vi "RunTimeMenuUI.vi"() -> ()   [LabVIEW 2015, in "RunTimeMenuItem.lvclass"]
uses:
  RunTimeMenuItem.lvclass
  <vilib>/NI/Configuration Framework/Node/NodeRef.ctl
  <vilib>/NI/Configuration Framework/Node/NISE_CEF_Node.lvclass
  <vilib>/NI/AMC/Message Queue.ctl
  <vilib>/NI/AMC/Message.ctl
  <vilib>/NI/Tools/Keyed Array/KeyedArray.ctl
  <vilib>/NI/Configuration Framework/Node/UserEventRef.ctl
  <vilib>/NI/Configuration Framework/Controls/EventCluster.ctl
  RunTimeMenuItem.lvclass/RunTimeMenuItem.ctl
  Read Run Time Menu Properties.vi
  Write Run Time Menu Properties.vi
  <vilib>/NI/AMC/Create Single Message.vi
  <vilib>/NI/AMC/Update Message Routing Info.vi
  <vilib>/NI/AMC/Send Message.vi
  <vilib>/NI/AMC/AMC.lvlib
  Configuration Tool.lvlib
  <vilib>/NI/Tools/Keyed Array/Tools_KeyedArray.lvlib
  <vilib>/NI/Configuration Framework/NISE_CEF_TreeControl.lvlib
panel:
  in  "Min # Of Children":u32
  in  "Dependency Behavior":enum16{"Static", "Dynamic"}(ring)
  in  "Behavior":enum16{"Nothing", "Open Front Panel"}(ring)
  in  "Position":enum16{"Centered", "Mouse Pointer"}(ring)
  in  "Execution":enum16{"silent", "modal", "floating", "default"}(ring)
  in  "Menu Item Type":enum16{"Action", "VI", "Separator", "Custom"}(ring)
  in  "Host Path to Dependency File":path
  in  "Host Path to Menu VI":path
  in  "Host Path to Custom Menu Item":path
  in  "GUID":string="9b525fa0-4d4a-4ec1-902b-bfeef88ebbcc"
  in  "Name":string
  in  "user event":T1
  in  "main queue":T2
  in  "node ref":T3
  # "General Settings"
  # "Advanced Settings"
  # "Dependency File Settings"
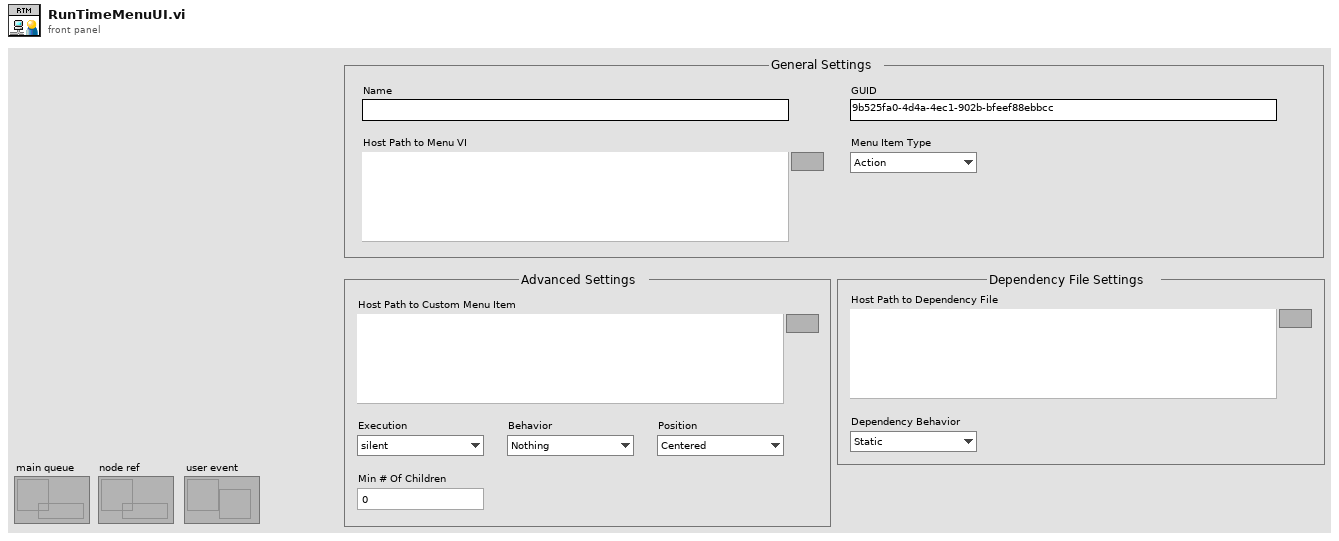
[diagram p1: front panel]
types:
  T1 = typedef "NISE_CEF_Node.lvclass/UserEventRef.ctl" = refnum<user-event>
  T2 = typedef "AMC.lvlib/Message Queue.ctl" = refnum<queue>
  T3 = typedef "NISE_CEF_Node.lvclass/NodeRef.ctl" = refnum<data-value>
  T4 = typedef "VeriStand Custom Device XML Parser.lvlib/RunTimeMenus Properties.ctl" = cluster{"GUID":string, "Execution":T5, "MinNrOfChilds":u32, "Name":string, "Item to Launch":T6, "Dependency":T7, "Custom Population":T6, "Menu Item Type":enum16{"Action", "VI", "Separator", "Custom"}, "Behavior":enum16{"Nothing", "Open Front Panel"}, "Position":enum16{"Centered", "Mouse Pointer"}}
  T5 = typedef "VeriStand Custom Device XML Parser.lvlib/Execution Types.ctl" = enum16{"silent", "modal", "floating", "default"}
  T6 = typedef "VeriStand Custom Device XML Parser.lvlib/Path Cluster.ctl" = cluster{"Path":path, "Path Type":enum16{"Absolute", "To Base", "To Common Doc Dir", "To Application Data Dir"}}
  T7 = typedef "VeriStand Custom Device XML Parser.lvlib/Dependency Properties.ctl" = cluster{"File Path Control":path, "Path Type":enum16{"Absolute", "To Base", "To Common Doc Dir", "To Application Data Dir"}, "Behavior":enum16{"Static", "Dynamic"}}
  T8 = enum16{"Absolute", "To Base", "To Common Doc Dir", "To Application Data Dir"}
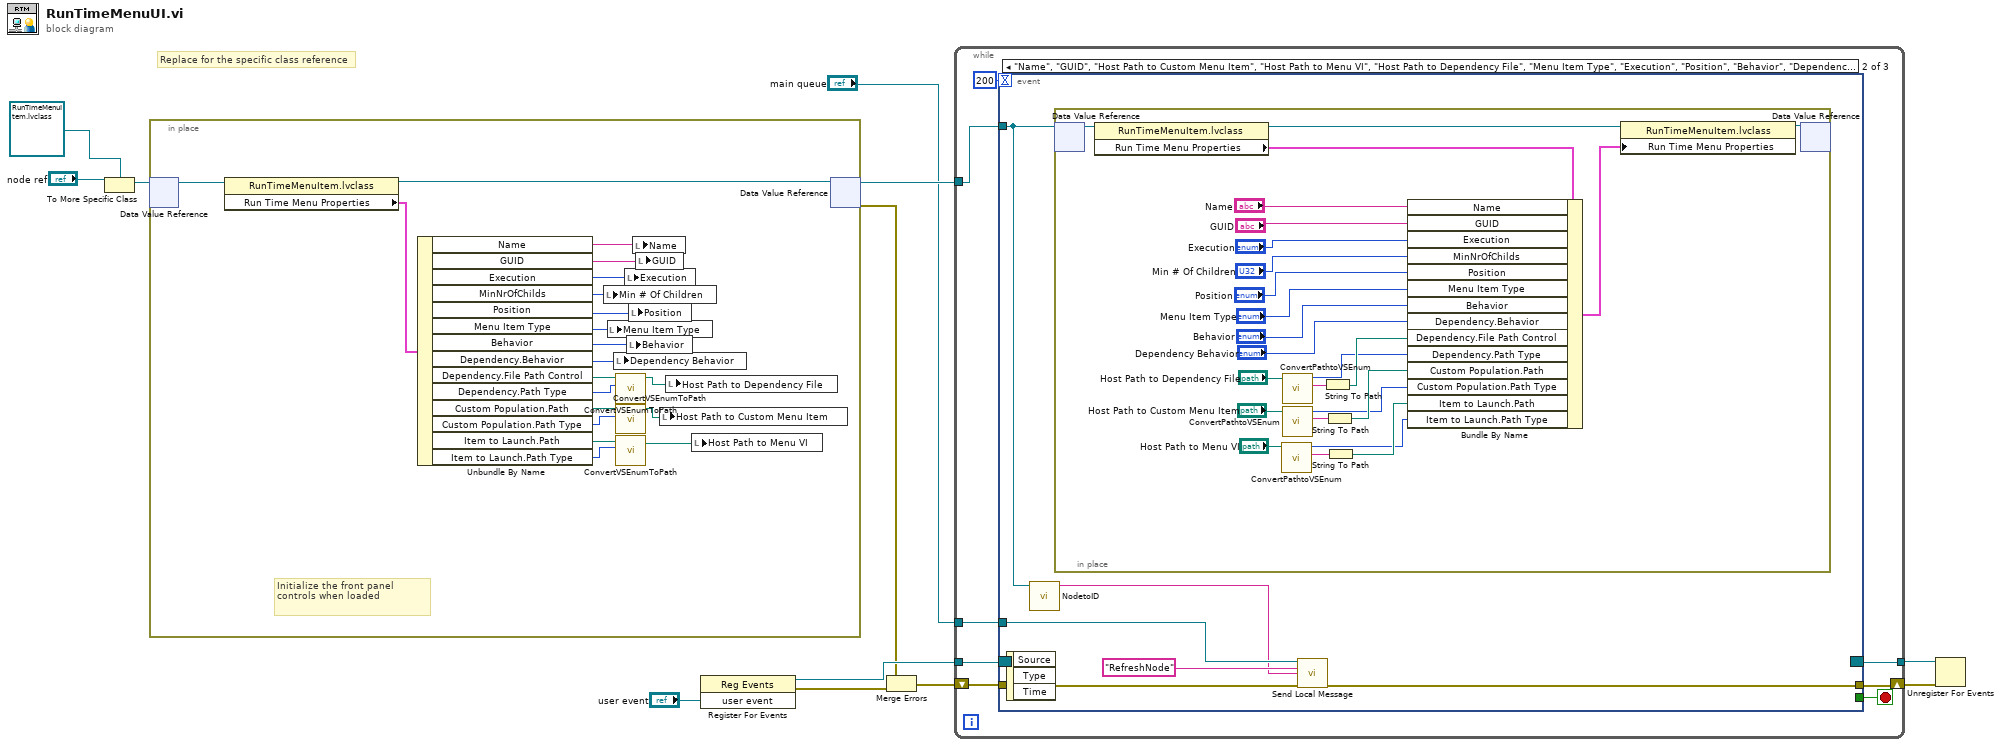
[diagram p0: block diagram]
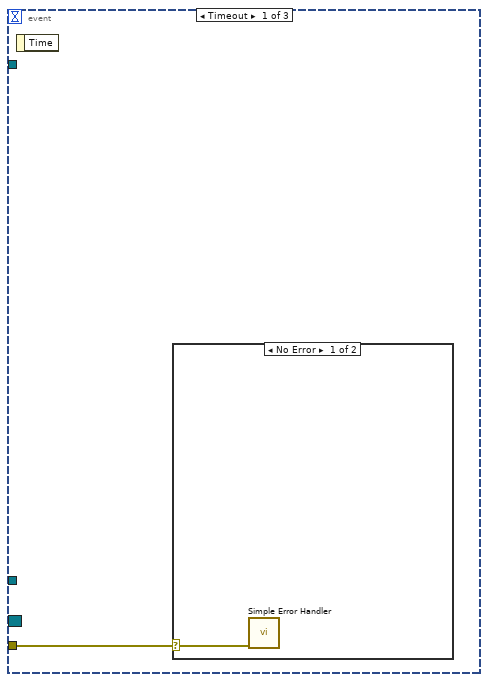
[diagram p2: hidden frame]
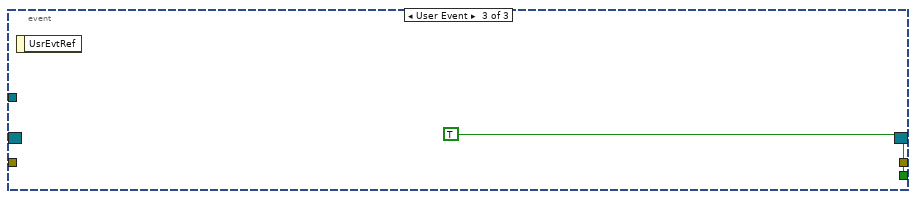
[diagram p4: hidden frame]
diagram:
  # "Replace for the specific class reference"
  n1 = To More Specific Class(target class=refnum<data-value> refnum ("data value reference"), reference="node ref") -> (specific class reference=w5:refnum<data-value>)  [unwired: 1 in, 1 out]
  n2 = in-place {
    # "Initialize the front panel controls when loaded"
    n3 = in-place-dvr #1(w5) -> (w32:refnum<class "RunTimeMenuItem.lvclass">)  [unwired: 1 out]
    n4 = property class="RunTimeMenuItem.lvclass"(reference=w32) -> (reference out=w31:refnum<class "RunTimeMenuItem.lvclass">, "Run Time Menu Properties"=w30:T4)  [unwired: 1 in, 1 out]
    n5 = Unbundle By Name(w30) -> ("Name"=w29:string, "GUID"=w28:string, "Execution"=w27:T5, "MinNrOfChilds"=w26:u32, "Position"=w25:enum16{"Centered", "Mouse Pointer"}, "Menu Item Type"=w24:enum16{"Action", "VI", "Separator", "Custom"}, "Behavior"=w23:enum16{"Nothing", "Open Front Panel"}, "Dependency.Behavior"=w22:enum16{"Static", "Dynamic"}, "Dependency.File Path Control"=w21:path, "Dependency.Path Type"=w20:T8, "Custom Population.Path"=w19:path, "Custom Population.Path Type"=w18:T8, "Item to Launch.Path"=w17:path, "Item to Launch.Path Type"=w16:T8)
    n6 = local write "Min # Of Children"(w26) -> ()
    n7 = local write "Menu Item Type"(w24) -> ()
    n8 = local write "Dependency Behavior"(w22) -> ()
    n9 = call "ConvertVSEnumToPath.vi"("Source.Path Type"=w20, "Path In"=w21) -> ("appended path"=w15:path)  [unwired: 9 in]
    n10 = call "ConvertVSEnumToPath.vi"("Source.Path Type"=w18, "Path In"=w19) -> ("appended path"=w14:path)  [unwired: 9 in]
    n11 = call "ConvertVSEnumToPath.vi"("Source.Path Type"=w16, "Path In"=w17) -> ("appended path"=w13:path)  [unwired: 9 in]
    n12 = local write "Execution"(w27) -> ()
    n13 = local write "Behavior"(w23) -> ()
    n14 = local write "Position"(w25) -> ()
    n15 = local write "Name"(w29) -> ()
    n16 = local write "GUID"(w28) -> ()
    n17 = local write "Host Path to Custom Menu Item"(w14) -> ()
    n18 = local write "Host Path to Dependency File"(w15) -> ()
    n19 = local write "Host Path to Menu VI"(w13) -> ()
    n20 = in-place-dvr #1(w31) -> (w12:refnum<data-value>, w2:errorcluster)
  }
  n21 = register-events("user event") -> (reference out=w9:refnum<event-registration>, error out=w3:errorcluster)  [unwired: 2 in]
  n22 = Merge Errors(w2, w3) -> (w1:errorcluster)
  n23 = while {
    tunnel: w12 -> [w40]
    tunnel: "main queue" -> [w39]
    tunnel: w9 -> [w37]
    tunnel: [w36] -> w8
    shift-right: [w34] -> w7
    shift-left: w1 -> [w33]
    stop <- w35 stop-if-true
    n24 = event shown="[1] \"Name\", \"GUID\", \"Host Path to Custom Menu Item\", \"Host Path to Menu VI\", \"Host Path to Dependency File\", \"Menu Item Type\", \"Execution\", \"Position\", \"Behavior\", \"Dependency Behavior\", \"Min # Of Children\": Value Change" {
      selector: w37 -> [_ _ _]
      dyn-events: [_ _ _] -> w36
      timeout: 200 -> [_ _ _]
      tunnel: w40 -> [_ w46 _]
      tunnel: w39 -> [_ w47 _]
      tunnel: [_ _ TRUE] -> w35
      tunnel: [_ w44 _] -> w34
      tunnel: w33 -> [w41 w43 _]
      event Timeout {
        n25 = event-data() -> ()  [unwired: 1 in, 1 out]
        n26 = case shown="No Error" w41 {
          selector: w41 -> [w42 _]
          frame No Error {
            n27 = call <vilib>:"Simple Error Handler.vi"("error in (no error)"=w42) -> ()  [unwired: 4 in, 5 out]
          }
          frame Error {
          }
        }
      }
      event "Name", "GUID", "Host Path to Custom Menu Item", "Host Path to Menu VI", "Host Path to Dependency File", "Menu Item Type", "Execution", "Position", "Behavior", "Dependency Behavior", "Min # Of Children": Value Change {
        n28 = event-data() -> ()  [unwired: 1 in, 3 out]
        n29 = call <vilib>:"NodetoID.vi"("node ref"=w46) -> ("ID"=w45:string)  [unwired: 9 in, 1 out]
        n30 = in-place {
          n31 = in-place-dvr #2(w46) -> (w71:refnum<class "RunTimeMenuItem.lvclass">)  [unwired: 1 out]
          n32 = property class="RunTimeMenuItem.lvclass"(reference=w71) -> (reference out=w70:refnum<class "RunTimeMenuItem.lvclass">, "Run Time Menu Properties"=w69:T4)  [unwired: 1 in, 1 out]
          n33 = call "ConvertPathtoVSEnum.vi"("Path In"="Host Path to Menu VI") -> ("Remaining Path"=w52:string, "VS Enum Out"=w50:T8)  [unwired: 9 in]
          n34 = call "ConvertPathtoVSEnum.vi"("Path In"="Host Path to Dependency File") -> ("Remaining Path"=w72:string, "VS Enum Out"=w58:T8)  [unwired: 9 in]
          n35 = call "ConvertPathtoVSEnum.vi"("Path In"="Host Path to Custom Menu Item") -> ("Remaining Path"=w56:string, "VS Enum Out"=w54:T8)  [unwired: 9 in]
          n36 = String To Path(string=w72) -> (path=w59:path)
          n37 = String To Path(string=w56) -> (path=w55:path)
          n38 = String To Path(string=w52) -> (path=w51:path)
          n39 = Bundle By Name(cluster=w69, "Name"="Name", "GUID"="GUID", "Execution"="Execution", "MinNrOfChilds"="Min # Of Children", "Position"="Position", "Menu Item Type"="Menu Item Type", "Behavior"="Behavior", "Dependency.Behavior"="Dependency Behavior", "Dependency.File Path Control"=w59, "Dependency.Path Type"=w58, "Custom Population.Path"=w55, "Custom Population.Path Type"=w54, "Item to Launch.Path"=w51, "Item to Launch.Path Type"=w50) -> (w49:T4)
          n40 = property class="RunTimeMenuItem.lvclass"(reference=w70, "Run Time Menu Properties"=w49) -> (reference out=w73:refnum<class "RunTimeMenuItem.lvclass">)  [unwired: 1 in, 1 out]
          n41 = in-place-dvr #2(w73) -> ()  [unwired: 2 out]
        }
        n42 = call <vilib>:"Send Local Message.vi"("message queue in"=w47, "message name"="RefreshNode" ("Message Name"), "message value"=w45, "error in"=w43) -> ("error out"=w44:errorcluster)  [unwired: 9 in, 2 out]
      }
      event User Event {
        n43 = event-data() -> ()  [unwired: 1 in, 1 out]
      }
    }
  }
  n44 = Unregister For Events(event registration refnum=w8, error in=w7) -> ()  [unwired: 1 out]
